vi "Select and Translate Tag.vi"(10 "Current Item":string="No-Outline") -> (2 "index of element":i32)   [LabVIEW 2021, in "Material SubVIs.lvlib"]
doc: "This VI provides backwards compatibility with the right-click option for the Boolean Type. Translates the old tags into the new options and selects the correct one if applicable.\n\n<b>Code Developed By:</b> +\nDaniel Coons +\nTechnology Service Corporation +\nwww.tsc.com/atcs"
uses:
  Material SubVIs.lvlib
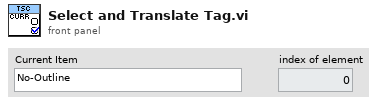
[diagram p1: front panel]
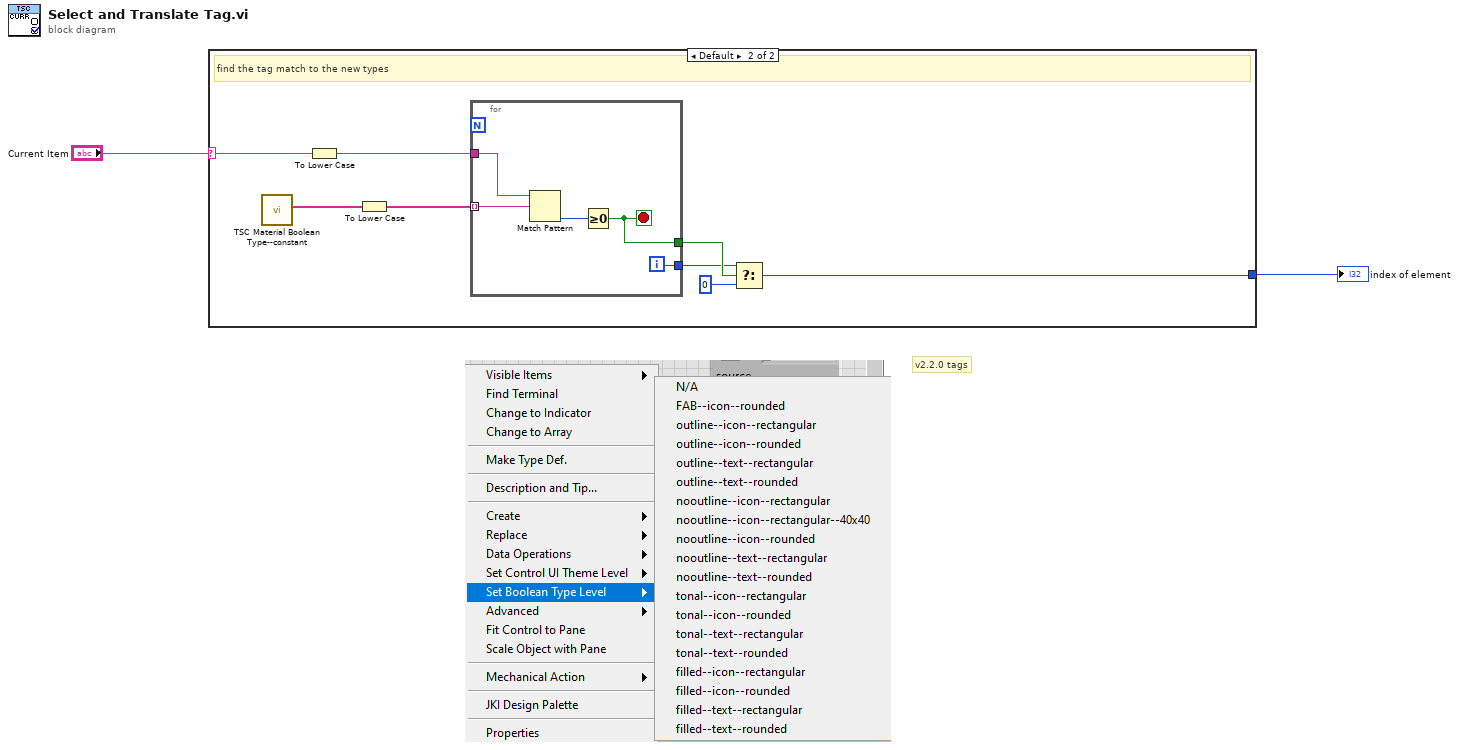
[diagram p0: block diagram]
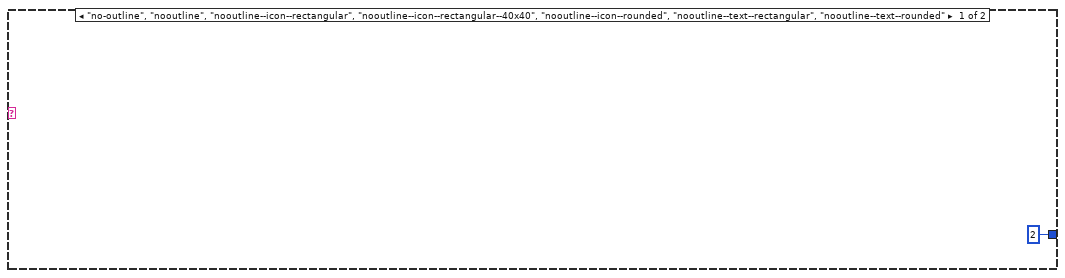
[diagram p2: hidden frame]
diagram:
  # "v2.2.0 tags"
  n1 = case shown="Default" "Current Item" {
    selector: "Current Item" -> [_ w4]
    tunnel: [2 ("f") w8] -> w2
    frame "no-outline", "nooutline", "nooutline--icon--rectangular", "nooutline--icon--rectangular--40x40", "nooutline--icon--rounded", "nooutline--text--rectangular", "nooutline--text--rounded" {
    }
    frame Default {
      # "find the tag match to the new types"
      n2 = call "TSC Material Boolean Type--constant.vi"() -> ("boolean types"=w11:string[])  [unwired: 11 in]
      n3 = To Lower Case(string=w4) -> (all lower case string=w10:string)
      n4 = To Lower Case(string=w11) -> (all lower case string=w9:string[])
      n5 = for {
        tunnel: w9 -> [w16] mode=indexing
        tunnel: w10 -> [w15]
        tunnel: [w13] -> w7
        tunnel: [w12] -> w6
        i -> [w12]
        stop <- w13 stop-if-true
        n6 = Match Pattern(string=w15, regular expression=w16) -> (offset past match=w14:i32)  [unwired: 1 in, 3 out]
        n7 = Greater Or Equal To 0?(x=w14) -> (x >= 0?=w13:bool)
      }
      n8 = Select(t=w6, s=w7, f=0) -> (s? t:f=w8:i32)
    }
  }
  "index of element" <- w2
